vi "Dashboard Build_Change Target Location.vi"(11 "Dashboard exe Path":path) -> ()   [LabVIEW 2020]
uses:
  <vilib>/Utility/config.llb/Read Key (String).vi
  <vilib>/Utility/config.llb/Write Key (String).vi
  <vilib>/Utility/config.llb/NI_LVConfig.lvlib
panel:
  out "Final string":string
  out "New Path":string
  out "Original Path":string
  out "Original  Stirng":string
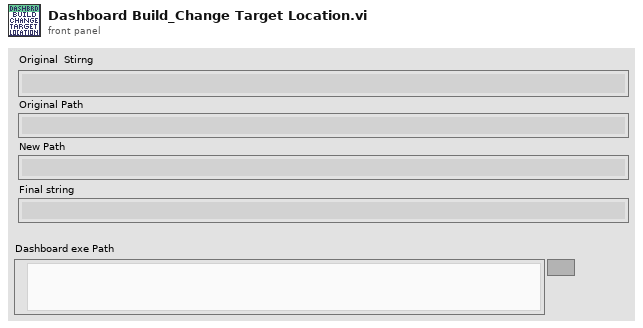
[diagram p1: front panel]
types:
  T1 = typedef "NI_LVConfig.lvlib/Config Data RefNum.ctl" = refnum<k1>
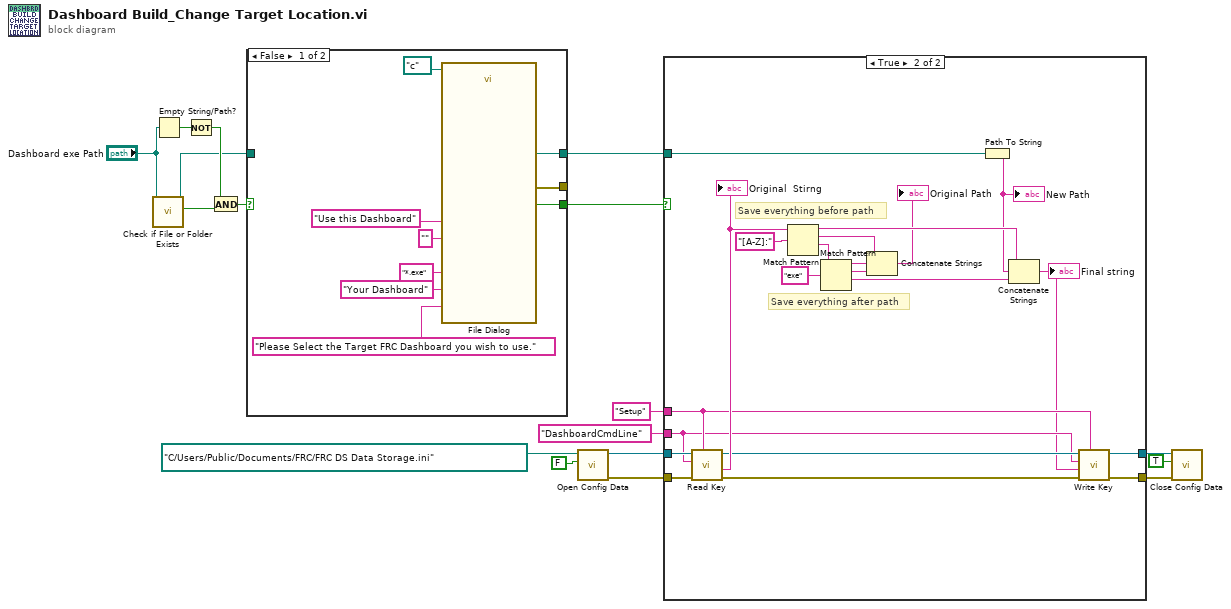
[diagram p0: block diagram]
diagram:
  n1 = call <vilib>:"Check if File or Folder Exists.vi"("path"="Dashboard exe Path") -> ("file or folder exists?"=w17:bool, "dup path"=w12:path)  [unwired: 8 in, 1 out]
  n2 = Empty String/Path?(string/path="Dashboard exe Path") -> (empty?=w16:bool)
  n3 = Not(x=w16) -> (.not. x?=w14:bool)
  n4 = And(x=w14, y=w17) -> (x .and. y?=w15:bool)
  n5 = case shown="False" w15 {
    selector: w15 -> [_ w27]
    tunnel: w12 -> [_ w28]
    tunnel: [w23 w27] -> w10
    tunnel: [w19 w28] -> w11
    tunnel: [w18 _] -> _
    frame False {
      n6 = call "File Dialog"("start path"=path "c:/", "prompt"="Please Select the Target FRC Dashboard you wish to use.", "button label"="Use this Dashboard", "default name"="", "pattern (all files)"="*.exe", "pattern label"="Your Dashboard") -> ("selected path"=w19:path, "exists"=w23:bool, "error out"=w18:errorcluster)  [unwired: 6 in, 1 out]
    }
    frame True {
    }
  }
  n7 = call <vilib>:"Open Config Data.vi"("create file if necessary (T)"=FALSE, "configuration file path"=path "C:/Users/Public/Documents/FRC/FRC DS Data Storage.ini" ("DS Data Storage.ini")) -> ("error out"=w6:errorcluster, "refnum"=w7:T1)  [unwired: 7 in, 1 out]
  n8 = case shown="True" w10 {
    tunnel: w11 -> [_ w41]
    tunnel: w7 -> [w29 w39]
    tunnel: w6 -> [w30 w38]
    tunnel: "Setup" ("section") -> [_ w33]
    tunnel: "DashboardCmdLine" ("section") -> [_ w32]
    tunnel: [w30 w36] -> w3
    tunnel: [w29 w34] -> w2
    frame False {
    }
    frame True {
      # "Save everything after path"
      # "Save everything before path"
      n9 = call-poly <vilib>:"Read Key.vi"("section"=w33, "error in (no error)"=w38, "key"=w32, "refnum"=w39) -> ("error out"=w37:errorcluster, "value"=w50:string, "refnum out"=w35:T1)  [unwired: 4 in, 1 out]
      "Original  Stirng" <- w50
      n10 = Match Pattern(string=w50, regular expression="[A-Z]:") -> (before substring=w48:string, match substring=w46:string, after substring=w44:string)  [unwired: 1 in, 1 out]
      n11 = Match Pattern(string=w44, regular expression="exe") -> (before substring=w43:string, match substring=w42:string, after substring=w47:string)  [unwired: 1 in, 1 out]
      n12 = Concatenate Strings(w46, w43, w42) -> (→"Original Path":string)
      n13 = Path To String(path=w41) -> (string=w40:string)
      "New Path" <- w40
      n14 = Concatenate Strings(w48, w40, w47) -> (w31:string)
      "Final string" <- w31
      n15 = call-poly <vilib>:"Write Key.vi"("section"=w33, "error in (no error)"=w37, "value"=w31, "key"=w32, "refnum"=w35) -> ("error out"=w36:errorcluster, "refnum out"=w34:T1)  [unwired: 4 in, 1 out]
    }
  }
  n16 = call <vilib>:"Close Config Data.vi"("error in (no error)"=w3, "write file if changed (T)"=TRUE, "refnum"=w2) -> ()  [unwired: 7 in, 2 out]
